vi "Motion Profile Right Drive Control.vi"(10 "Start Motion Profile?":bool, 11 "Cluster in":T11) -> (3 "Cluster out":T11)   [LabVIEW 2018]
uses:
  <vilib>/Rock Robotics/WPI/Joystick/WPI_JoystickDevRef.ctl
  <vilib>/Rock Robotics/WPI/Joystick/WPI_JoystickDeviceEnum.ctl
  <vilib>/Rock Robotics/WPI/DriverStation/WPI_DriverStationRobotMode2.ctl
  <vilib>/Rock Robotics/WPI/RobotDrive/WPI_RobotDriveDevRef.ctl
  <vilib>/Rock Robotics/WPI/MotorControl/WPI_MotorControlDeviceRef.ctl
  <vilib>/Rock Robotics/WPI/MotorControl/WPI_MotorControlType.ctl
  <vilib>/Rock Robotics/SystemInterfaces/DIO/FPGA_DIOPWMChannel.ctl
  <vilib>/Rock Robotics/WPI/PWM/WPI_PWMDeadband.ctl
  <vilib>/Rock Robotics/SystemInterfaces/DIO/FPGA_DIOChannel.ctl
  Vision States.ctl
  <vilib>/Rock Robotics/WPI/ThirdParty/Phoenix-LabVIEW/Motor Controller/Controls/CTRE_Phoenix_MotorControl_MotionProfileControlMode.ctl
  Robot Global Data.vi
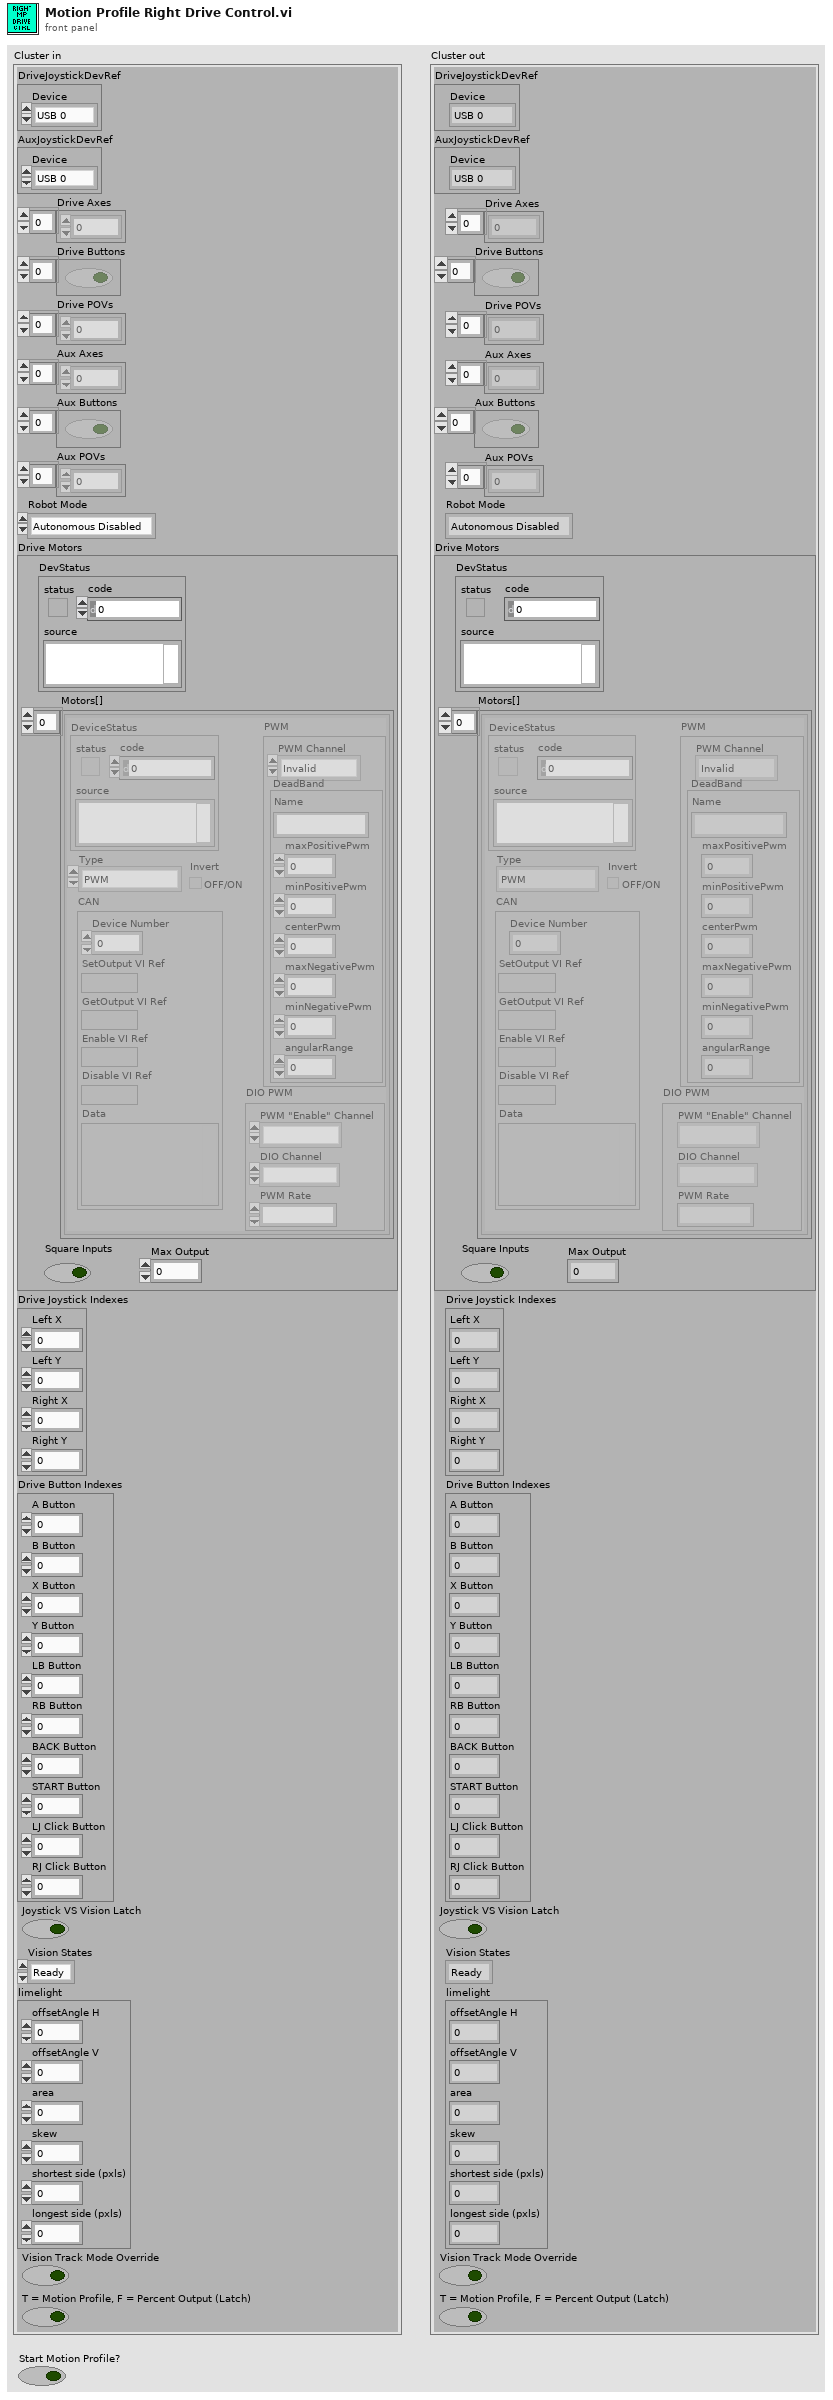
[diagram p1: front panel]
types:
  T1 = typedef "WPI_JoystickDevRef.ctl" = cluster{"Device":T2}
  T2 = typedef "WPI_JoystickDeviceEnum.ctl" = enum16{"USB 0", "USB 1", "USB 2", "USB 3", "USB 4", "USB 5"}
  T3 = typedef "WPI_DriverStationRobotMode2.ctl" = enum16{"Autonomous Disabled", "Autonomous Enabled", "Teleop Disabled", "Teleop Enabled", "Disconnected", "Finish", "Test Disabled", "Test Enabled", "Emergency Stopped"}
  T4 = typedef "WPI_RobotDriveDevRef.ctl" = cluster{"DevStatus":errorcluster, "Motors[]":T5[], "Square Inputs":bool, "Max Output":dbl}
  T5 = typedef "WPI_MotorControlDeviceRef.ctl" = cluster{"DeviceStatus":errorcluster, "Type":T6, "PWM":cluster{"PWM Channel":T7, "DeadBand":T8}, "CAN":cluster{"Device Number":u8, "SetOutput VI Ref":variant, "GetOutput VI Ref":variant, "Enable VI Ref":variant, "Disable VI Ref":variant, "Data":variant}, "Invert":bool, "DIO PWM":cluster{"PWM \"Enable\" Channel":T7, "DIOChannel":T9, "PWM Rate":dbl}}
  T6 = typedef "WPI_MotorControlType.ctl" = enum16{"PWM", "CAN", "DIO PWM"}
  T7 = typedef "FPGA_DIOPWMChannel.ctl" = enum8{"PWM 0", "PWM 1", "PWM 2", "PWM 3", "PWM 4", "PWM 5", "PWM 6", "PWM 7", "PWM 8", "PWM 9", "PWM MXP 0", "PWM MXP 1", "PWM MXP 2", "PWM MXP 3", "PWM MXP 4", "PWM MXP 5", "PWM MXP 6", "PWM MXP 7", "PWM MXP 8", "PWM MXP 9", "Invalid"}
  T8 = typedef "WPI_PWMDeadband.ctl" = cluster{"Name":string, "maxPositivePwm":i32, "minPositivePwm":i32, "centerPwm":i32, "maxNegativePwm":i32, "minNegativePwm":i32, "angularRange":u16}
  T9 = typedef "FPGA_DIOChannel.ctl" = enum8{"DIO 0", "DIO 1", "DIO 2", "DIO 3", "DIO 4", "DIO 5", "DIO 6", "DIO 7", "DIO 8", "DIO 9", "DIO MXP 0", "DIO MXP 1", "DIO MXP 2", "DIO MXP 3", "DIO MXP 4", "DIO MXP 5", "DIO MXP 6", "DIO MXP 7", "DIO MXP 8", "DIO MXP 9", "DIO MXP 10", "DIO MXP 11", "DIO MXP 12", "DIO MXP 13", "DIO MXP 14", "DIO MXP 15", "SPI Port CS1", "SPI Port CS2", "SPI Port CS3", "SPI Port MISO", "SPI Port MOSI", "Invalid"}
  T10 = typedef "Vision States.ctl" = enum16{"Ready", "Forward Until Target at Edge", "Vision Track"}
  T11 = cluster{"DriveJoystickDevRef":T1, "AuxJoystickDevRef":T1, "Drive Axes":dbl[], "Drive Buttons":bool[], "Drive POVs":i16[], "Aux Axes":dbl[], "Aux Buttons":bool[], "Aux POVs":i16[], "Robot Mode":T3, "Drive Motors":T4, "Drive Joystick Indexes":cluster{"Left X":i32, "Left Y":i32, "Right X":i32, "Right Y":i32}, "Drive Button Indexes":cluster{"A Button":i32, "B Button":i32, "X Button":i32, "Y Button":i32, "LB Button":i32, "RB Button":i32, "BACK Button":i32, "START Button":i32, "LJ Click Button":i32, "RJ Click Button":i32}, "Joystick VS Vision Latch":bool, "Vision States":T10, "limelight":cluster{"offsetAngle H":dbl, "offsetAngle V":dbl, "area":dbl, "skew":dbl, "shortest side (pxls)":dbl, "longest side (pxls)":dbl}, "Vision Track Mode Override":bool, "T = Motion Profile, F = Percent Output (Latch)":bool}
  T12 = cluster{"Top Buffer Remaining":i32, "Top Buffer Count":i32, "Bottom Buffer Count":i32, "Has Underrun?":bool, "Is Underrun?":bool, "Active Point Valid?":bool, "Is Last?":bool, "Profile Slot Select 0":i32, "Output Enable":i32, "Time Duration (ms)":i32, "Profile Slot Select 1":i32}
  T13 = typedef "CTRE_Phoenix_MotorControl_MotionProfileControlMode.ctl" = u16
  T14 = typedef "CTRE_Phoenix_MotorControl_BufferedTrajectoryPointStream_DeviceRef.ctl" = cluster{"Handle":u64, "Library Path":path}
  T15 = cluster{"Mot Prof Active Velocity":dbl, "Mot Prof Active Position":dbl, "Mot Prof  Is Under Run":bool, "Mot Prof  Has Under Run":bool, "Mot Prof Active Is Last":bool, "Mot Prof Active Is Valid":bool, "Top Mot Prof Count":i32, "Btm Mot Prof Count":i32, "Is Motion Profile Finished?":bool}
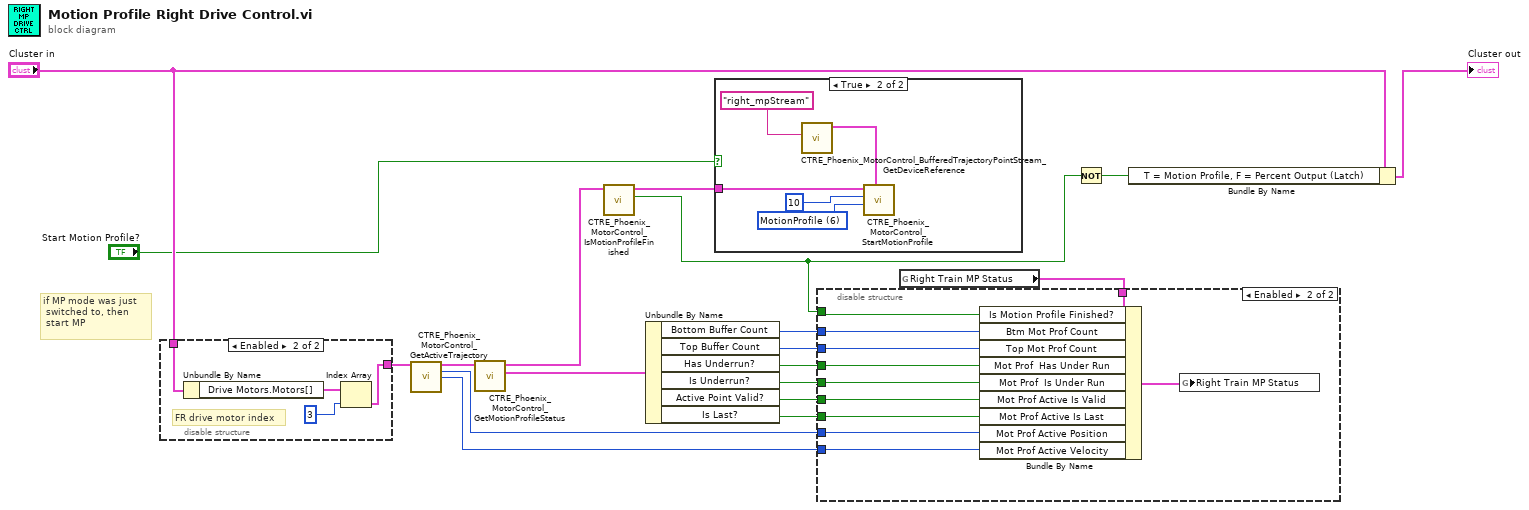
[diagram p0: block diagram]
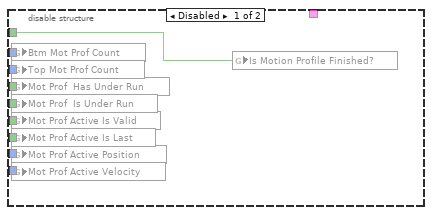
[diagram p2: hidden frame]
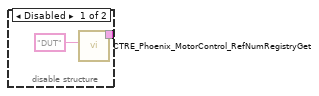
[diagram p3: hidden frame]
diagram:
  # "if MP mode was just\n switched to, then\n start MP"
  n1 = disable-structure shown="Enabled" {
    disable-tunnel: [w21 w24] -> w15
    disable-tunnel: "Cluster in" -> [_ w25]
    frame Disabled {
      n2 = call <vilib>:"CTRE_Phoenix_MotorControl_RefNumRegistryGet.vi"("refnum name"="DUT") -> ("PhoenixMotorControlDevRef"=w21:T5)  [unwired: 9 in, 1 out]
    }
    frame Enabled {
      # "FR drive motor index"
      n3 = Unbundle By Name(w25) -> ("Drive Motors.Motors[]"=w23:T5[])
      n4 = Index Array(array=w23, index=3) -> (element=w24:T5)
    }
  }
  n5 = call <vilib>:"CTRE_Phoenix_MotorControl_GetActiveTrajectory.vi"("PhoenixMotorControlDevRef"=w15) -> ("PhoenixMotorControlDevRef"=w13:T5, "Position (Sensor Units)"=w2:i32, "Velocity (Sensor Units per 100 ms)"=w1:i32)  [unwired: 10 in, 2 out]
  n6 = call <vilib>:"CTRE_Phoenix_MotorControl_GetMotionProfileStatus.vi"("PhoenixMotorControlDevRef"=w13) -> ("Motion Profile Status"=w14:T12, "PhoenixMotorControlDevRef"=w12:T5)  [unwired: 8 in, 1 out]
  n7 = call <vilib>:"CTRE_Phoenix_MotorControl_IsMotionProfileFinished.vi"("PhoenixMotorControlDevRef"=w12) -> ("Is Motion Profile Finished?"=w9:bool, "PhoenixMotorControlDevRef"=w11:T5)  [unwired: 8 in, 1 out]
  n8 = Unbundle By Name(w14) -> ("Bottom Buffer Count"=w8:i32, "Top Buffer Count"=w7:i32, "Has Underrun?"=w6:bool, "Is Underrun?"=w5:bool, "Active Point Valid?"=w4:bool, "Is Last?"=w3:bool)
  n9 = case shown="True" "Start Motion Profile?" {
    tunnel: w11 -> [_ w30]
    frame False {
    }
    frame True {
      w29 = T13 6 items=["MotionProfile"=6, "MotionProfileArc"=10] ("Control Mode")
      n10 = call <vilib>:"CTRE_Phoenix_MotorControl_BufferedTrajectoryPointStream_GetDeviceReference.vi"("refnum name"="right_mpStream") -> ("BufferedTrajectoryPointStream_DevRef"=w26:T14)  [unwired: 9 in, 1 out]
      n11 = call <vilib>:"CTRE_Phoenix_MotorControl_StartMotionProfile.vi"("BufferedTrajectoryPointStream_DevRef"=w26, "Control Mode"=w29, "minBufferedPts"=u32 10, "PhoenixMotorControlDevRef"=w30) -> ()  [unwired: 6 in, 2 out]
    }
  }
  n12 = global read "Robot Global Data.vi" "Right Train MP Status"() -> (w10:T15)
  n13 = disable-structure shown="Enabled" {
    disable-tunnel: w1 -> [w39 w47]
    disable-tunnel: w2 -> [w38 w48]
    disable-tunnel: w3 -> [w37 w41]
    disable-tunnel: w4 -> [w36 w42]
    disable-tunnel: w5 -> [w35 w43]
    disable-tunnel: w6 -> [w34 w44]
    disable-tunnel: w7 -> [w33 w49]
    disable-tunnel: w8 -> [w32 w50]
    disable-tunnel: w9 -> [w31 w46]
    disable-tunnel: w10 -> [_ w45]
    frame Disabled {
      n14 = global write "Robot Global Data.vi" "Btm Mot Prof Count"(w32) -> ()
      n15 = global write "Robot Global Data.vi" "Top Mot Prof Count"(w33) -> ()
      n16 = global write "Robot Global Data.vi" "Mot Prof  Has Under Run"(w34) -> ()
      n17 = global write "Robot Global Data.vi" "Mot Prof  Is Under Run"(w35) -> ()
      n18 = global write "Robot Global Data.vi" "Mot Prof Active Is Valid"(w36) -> ()
      n19 = global write "Robot Global Data.vi" "Mot Prof Active Is Last"(w37) -> ()
      n20 = global write "Robot Global Data.vi" "Mot Prof Active Position"(w38) -> ()
      n21 = global write "Robot Global Data.vi" "Mot Prof Active Velocity"(w39) -> ()
      n22 = global write "Robot Global Data.vi" "Is Motion Profile Finished?"(w31) -> ()
    }
    frame Enabled {
      n23 = Bundle By Name(cluster=w45, "Is Motion Profile Finished?"=w46, "Btm Mot Prof Count"=w50, "Top Mot Prof Count"=w49, "Mot Prof  Has Under Run"=w44, "Mot Prof  Is Under Run"=w43, "Mot Prof Active Is Valid"=w42, "Mot Prof Active Is Last"=w41, "Mot Prof Active Position"=w48, "Mot Prof Active Velocity"=w47) -> (w40:T15)
      n24 = global write "Robot Global Data.vi" "Right Train MP Status"(w40) -> ()
    }
  }
  n25 = Not(x=w9) -> (.not. x?=w17:bool)
  n26 = Bundle By Name(cluster="Cluster in", "T = Motion Profile, F = Percent Output (Latch)"=w17) -> (→"Cluster out":T11)
